vi "piezo2USBWrite.vi"(1 "mode":u16(ring) items=["fractional", "voltage (V)", "position (um)"], 2 "position":dbl) -> ()   [LabVIEW 2017]
uses:
  globalDevices.vi
  Piezo/lvlib/Madlib.lvlib
panel:
  out "function return":i32
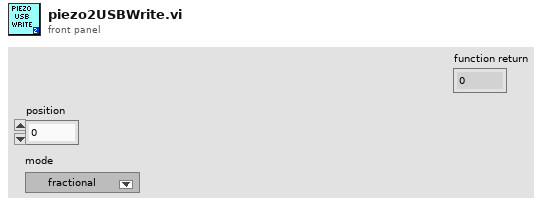
[diagram p1: front panel]
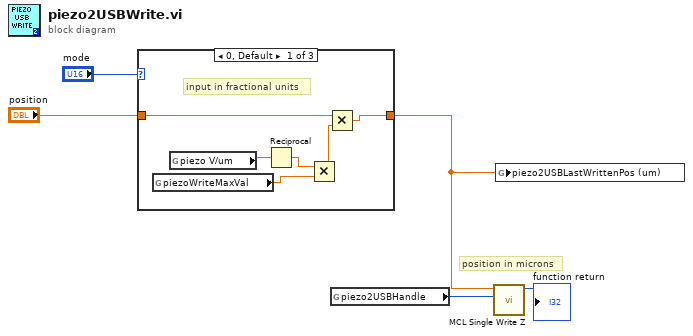
[diagram p0: block diagram]
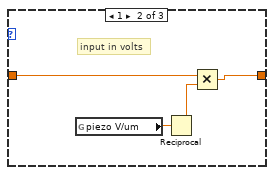
[diagram p2: hidden frame]
diagram:
  # "position in microns"
  n1 = case shown="0, Default" "mode" {
    tunnel: "position" -> [w11 w15 w16]
    tunnel: [w10 w14 w16] -> w2
    frame 0, Default {
      # "input in fractional units"
      n2 = global read "globalDevices.vi" "piezoWriteMaxVal"() -> (w9:dbl)
      n3 = global read "globalDevices.vi" "piezo V/um"() -> (w8:dbl)
      n4 = Reciprocal(x=w8) -> (1/x=w7:dbl)
      n5 = Multiply(x=w7, y=w9) -> (x*y=w6:dbl)
      n6 = Multiply(x=w11, y=w6) -> (x*y=w10:dbl)
    }
    frame 1 {
      # "input in volts"
      n7 = global read "globalDevices.vi" "piezo V/um"() -> (w13:dbl)
      n8 = Reciprocal(x=w13) -> (1/x=w12:dbl)
      n9 = Multiply(x=w15, y=w12) -> (x*y=w14:dbl)
    }
    frame 2 {
      # "input in microns"
    }
  }
  n10 = global read "globalDevices.vi" "piezo2USBHandle"() -> (w5:i32)
  n11 = call "MCL Single Write Z.vi"("handle"=w5, "position"=w2) -> ("function return"=→"function return":i32)  [unwired: 9 in]
  n12 = global write "globalDevices.vi" "piezo2USBLastWrittenPos (um)"(w2) -> ()
